vi "Write.vi"(8 "error in (no error)":errorcluster, 10 "Boolean":T1, 11 "Local Bus_DBL in":refnum<class "Fault-Injection_U32.lvclass">) -> (0 "error out":errorcluster, 3 "Local Bus_DBL out":refnum<class "Fault-Injection_U32.lvclass">)   [LabVIEW 2021, in "Fault-Injection_U32.lvclass"]
uses:
  Fault-Injection_U32.lvclass
  Fault-Injection_U32.lvclass/Fault-Injection_U32.ctl
  <vilib>/TSA/Abstract Data Classes/Abs_Types/U32 Integer/Abs_U32 Integer.lvclass
  Support/Value Type.ctl
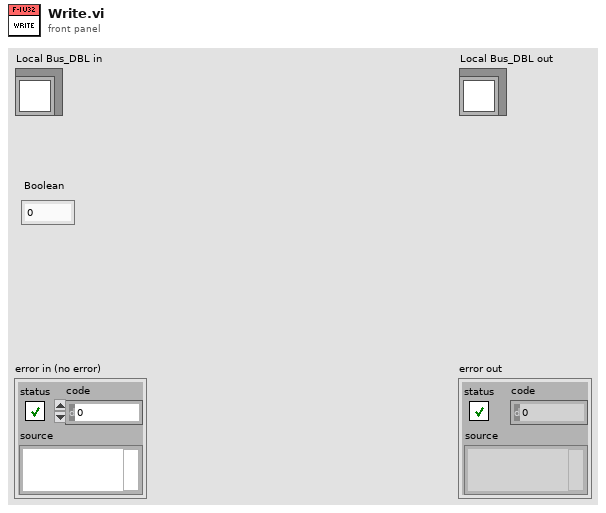
[diagram p1: front panel]
types:
  T1 = typedef "Fault-Injection_U32.lvclass/Value Type.ctl" = u32
  T2 = typedef "Fault-Injection_U32.lvclass/DVR Type.ctl" = cluster{"Enable":bool, "Injected Value":T1, "Value":T3}
  T3 = typedef "Fault-Injection_U32.lvclass/Abs Class Type.ctl" = refnum<class "Abs_U32 Integer.lvclass">
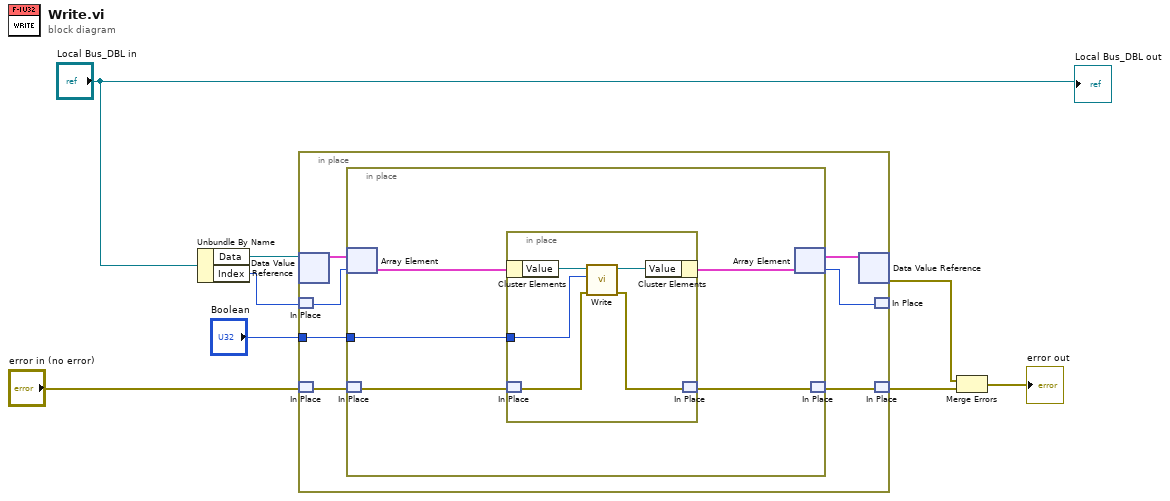
[diagram p0: block diagram]
diagram:
  n1 = Unbundle By Name("Local Bus_DBL in") -> ("Data"=w8:refnum<data-value>, "Index"=w7:i32)
  n2 = in-place {
    in-place-border: "Boolean" -> [w9]
    n3 = in-place-dvr #1(w8) -> (w15:T2[])  [unwired: 1 out]
    n4 = in-place-match #2(w7) -> (w13:i32)
    n5 = in-place-match #3("error in (no error)") -> (w11:errorcluster)
    n6 = in-place {
      in-place-border: w9 -> [w16]
      n7 = in-place-array #4(w15, w13) -> (w17:T2)
      n8 = in-place-match #5(w11) -> (w19:errorcluster)
      n9 = in-place {
        in-place-border: w16 -> [w21]
        n10 = in-place-cluster #6(w17) -> ("Value"=w22:T3)
        n11 = in-place-match #7(w19) -> (w24:errorcluster)
        n12 = call-dynamic "Write.vi"("error in (no error)"=w24, "Value"=w21, "Double Float.lvclass_340760 in"=w22) -> ("error out"=w23:errorcluster, "Double Float.lvclass_340760 out"=w25:T3)  [unwired: 7 in]
        n13 = in-place-cluster #6("Value"=w25) -> (w20:T2)
        n14 = in-place-match #7(w23) -> (w18:errorcluster)
      }
      n15 = in-place-array #4(w20) -> (w14:T2[], w12:i32)
      n16 = in-place-match #5(w18) -> (w10:errorcluster)
    }
    n17 = in-place-dvr #1(w14) -> (w5:errorcluster)  [unwired: 1 out]
    n18 = in-place-match #2(w12) -> ()  [unwired: 1 out]
    n19 = in-place-match #3(w10) -> (w6:errorcluster)
  }
  n20 = Merge Errors(w5, w6) -> (→"error out":errorcluster)
  "Local Bus_DBL out" <- "Local Bus_DBL in"
